vi "Pre Launch Init.vi"(11 "Instruments in":refnum<class "Instruments.lvclass">) -> (0 "error out":errorcluster, 3 "Instruments out":refnum<class "Instruments.lvclass">)   [LabVIEW 2023, in "Instruments.lvlib" / "Instruments.lvclass"]
uses:
  Library/Instruments.lvclass
  C:/Users/Public/Documents/Development/builds/Engine/Actor Framework.lvlibp/1abvi3w/vi.lib/ActorFramework/Actor/Actor.lvclass
  C:/Users/Public/Documents/Development/builds/Engine/Engine.lvlibp/Project/Engine.lvclass
  builds/Engine/Actor Framework.lvlibp/1abvi3w/vi.lib/ActorFramework/Actor/Read Actor Label.vi
  builds/Engine/Engine.lvlibp/Accessors/Read Directory.vi
  builds/Tools/Config.lvlibp/Config.lvclass
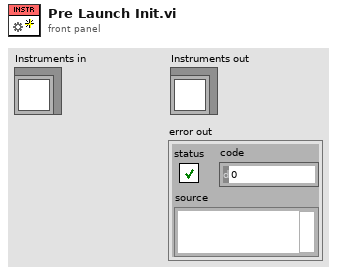
[diagram p1: front panel]
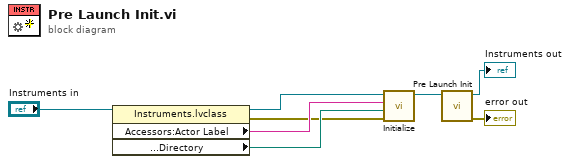
[diagram p0: block diagram]
diagram:
  n1 = property class="Instruments.lvclass"(reference="Instruments in") -> (reference out=w4:refnum<class "Instruments.lvclass">, error out=w3:errorcluster, "Accessors:Actor Label"=w5:string, "Accessors:Application:Information:Directory"=w6:path)  [unwired: 1 in]
  n2 = call-dynamic "Initialize.vi"("error in"=w3, "Path"=w6, "Device"=w5, "Instruments in"=w4) -> ("Instruments out"=w1:refnum<class "Instruments.lvclass">)  [unwired: 6 in, 1 out]
  n3 = call-parent "Pre Launch Init.vi"("Engine_Tools in"=w1) -> ("error out"=→"error out":errorcluster, "Engine_Tools out"=→"Instruments out":refnum<class "Instruments.lvclass">)  [unwired: 9 in]
